vi "Actor Core.vi"(8 "error in":errorcluster, 11 "CS++DCPwrGui.lvclass":refnum<class "CS++FgenGui.lvclass">) -> (0 "error out":errorcluster, 3 "Actor out":refnum<class "Actor.lvclass">)   [LabVIEW 2013, in "CS++FgenGui.lvlib" / "CS++FgenGui.lvclass"]
doc: "(<B>Filename</B>: Actor Framework.lvlib:Actor.lvclass:Actor Core.vi)\n\nReceives messages to the actor, reacts to them, and initiates any error handling that may shut the actor down.\n\nDescendant classes may override this VI to append parallel tasks for the actor to complete while it handles messages. Overrides use the Call Parent Method node."
uses:
  CS++FgenGui.lvclass
  <vilib>/ActorFramework/Actor/Actor.lvclass
  Core/Classes/CS++ProcessVariables/ProcessVariable/PV.lvclass
  Core/Actors/CS++SVMonitor/CS++SVMonitor.lvclass
  CS++DCPwrGui Messages/Update PV Msg/Update PV Msg.lvclass
  Core/Actors/CS++BaseActor/CS++BaseActor.lvclass/CS++BaseActor.ctl
  <vilib>/ActorFramework/Actor/Actor.lvclass/Actor.ctl
  <vilib>/ActorFramework/Message Enqueuer/Message Enqueuer.lvclass/Message Enqueuer.ctl
  Core/Actors/CS++DeviceGUIActor/CS++DeviceGUIActor.lvclass/CS++DeviceGUIActor.ctl
  Core/Classes/CS++BaseClasses/Factory/CS++Factory.lvclass
  Core/Actors/CS++PVMonitor/CS++PVMonitor.lvclass/CS++PVMonitor.ctl
  Core/Actors/CS++GUIActor/CS++GUIActor.lvclass/CS++GUIActor.ctl
  Core/Actors/CS++PVMonitor Messages/Register PVs Msg/Register PVs Msg.lvclass/Register PVs Msg.ctl
  CS++FgenGui.lvclass/CS++FgenGui.ctl
  Core/Actors/CS++DeviceGUIActor/CS++DeviceGUIActor.lvclass
  Core/Classes/CS++ProcessVariables/ProcessVariable/PV.lvclass/PV.ctl
  CS++DCPwr Messages/Configure Output Enable Msg/Configure Output Enable Msg.lvclass/Configure Output Enable Msg.ctl
  CS++DCPwr Messages/Configure Output Range Msg/Configure Output Range Msg.lvclass/Configure Output Range Msg.ctl
  CS++DCPwr Messages/Configure Current Limit Msg/Configure Current Limit Msg.lvclass/Configure Current Limit Msg.ctl
  CS++DCPwr Messages/Query Max Voltage Level Msg/Query Max Voltage Level Msg.lvclass/Query Max Voltage Level Msg.ctl
  CS++DCPwr Messages/Configure OVP Msg/Configure OVP Msg.lvclass/Configure OVP Msg.ctl
  CS++DCPwr Messages/Query Max Current Limit Msg/Query Max Current Limit Msg.lvclass/Query Max Current Limit Msg.ctl
  CS++DCPwr Messages/Configure Trigger Source [TRG] Msg/Configure Trigger Source [TRG] Msg.lvclass/Configure Trigger Source [TRG] Msg.ctl
  CS++DCPwr Messages/Configure Triggered Voltage Level [TRG] Msg/Configure Triggered Voltage Level [TRG] Msg.lvclass/Configure Triggered Voltage Level [TRG] Msg.ctl
  CS++DCPwr Messages/Configure Triggered Current Limit [TRG] Msg/Configure Triggered Current Limit [TRG] Msg.lvclass/Configure Triggered Current Limit [TRG] Msg.ctl
  CS++DCPwr Messages/Configure Voltage Level Msg/Configure Voltage Level Msg.lvclass/Configure Voltage Level Msg.ctl
  Core/Actors/CS++DeviceGUIActor/Read Resource Name.vi
  Core/Actors/CS++DeviceGUIActor/Read Driver Revision.vi
  Core/Actors/CS++DeviceGUIActor/Read Firmware Revision.vi
  Core/Actors/CS++DeviceGUIActor/Read Self-Test Result Code.vi
  Core/Actors/CS++DeviceGUIActor/Read Self-Test Result Message.vi
  Core/Classes/CS++ProcessVariables/ProcessVariable/Read Data.vi
  Core/Classes/CS++ProcessVariables/ProcessVariable/Read Timestamp.vi
  <vilib>/ActorFramework/Message Enqueuer/Init from Existing Queue.vi
  <vilib>/ActorFramework/Message Enqueuer/Enqueue.vi
  <vilib>/ActorFramework/Message Priority Queue/Priority Enqueue.vi
  <vilib>/ActorFramework/Message Enqueuer/Message Enqueuer.lvclass
  Core/Actors/CS++PVMonitor Messages/CS++PVUpdate Msg/CS++PVUpdate Msg.lvclass
  Core/Actors/CS++PVMonitor Messages/Register PVs Msg/Register PVs Msg.lvclass
  <vilib>/ActorFramework/Stop Msg/Stop Msg.lvclass
  CS++DCPwr Messages/Configure Output Enable Msg/Configure Output Enable Msg.lvclass
  CS++DCPwr Messages/Configure Output Range Msg/Configure Output Range Msg.lvclass
  CS++DCPwr Messages/Configure Current Limit Msg/Configure Current Limit Msg.lvclass
  CS++DCPwr Messages/Query Max Voltage Level Msg/Query Max Voltage Level Msg.lvclass
  CS++DCPwr Messages/Configure OVP Msg/Configure OVP Msg.lvclass
  CS++DCPwr Messages/Query Max Current Limit Msg/Query Max Current Limit Msg.lvclass
  CS++DCPwr Messages/Configure Trigger Source [TRG] Msg/Configure Trigger Source [TRG] Msg.lvclass
  CS++DCPwr Messages/Configure Triggered Voltage Level [TRG] Msg/Configure Triggered Voltage Level [TRG] Msg.lvclass
  CS++DCPwr Messages/Configure Triggered Current Limit [TRG] Msg/Configure Triggered Current Limit [TRG] Msg.lvclass
  CS++DCPwr Messages/Configure Voltage Level Msg/Configure Voltage Level Msg.lvclass
  CS++DCPwr Messages/Initiate [TRG] Msg/Initiate [TRG] Msg.lvclass
  CS++DCPwr Messages/Send Software Trigger [SWT] Msg/Send Software Trigger [SWT] Msg.lvclass
  CS++DCPwr Messages/Abort [TRG] Msg/Abort [TRG] Msg.lvclass
  Core/Actors/CS++BaseActor/CS++BaseActor.lvclass
  Core/Actors/CS++GUIActor/CS++GUIActor.lvclass
  Core/Actors/CS++PVMonitor/CS++PVMonitor.lvclass
panel:
  in  "Tab Control":enum32{"Info", "Configuration", "Output"}(tab)
  out "Actor Name":string
  out "Driver Revision":string
  out "Firmware Revision":string
  out "Self-Test Result Code":i32
  out "Self-Test Result Message":string
  out "Resource Name":string
  out "Number Of Channels":i32
  in  "Configuration Settings":string[][](table)
  in  "Initiate":bool
  in  "Send Software Trigger":bool
  in  "Abort":bool
  out "Timestamp":timestamp
  in  "Stop Button":bool
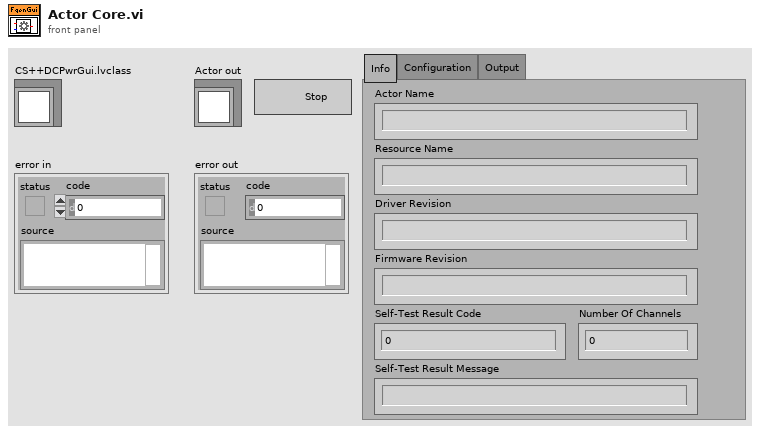
[diagram p1: front panel]
types:
  T1 = enum32{"Invalid", "Standard", "Closed", "Hidden", "Minimized", "Maximized"}
  T2 = cluster{string, "CS++FgenGui.lvlib:Update PV Msg.lvclass":refnum<class "Update PV Msg.lvclass">}
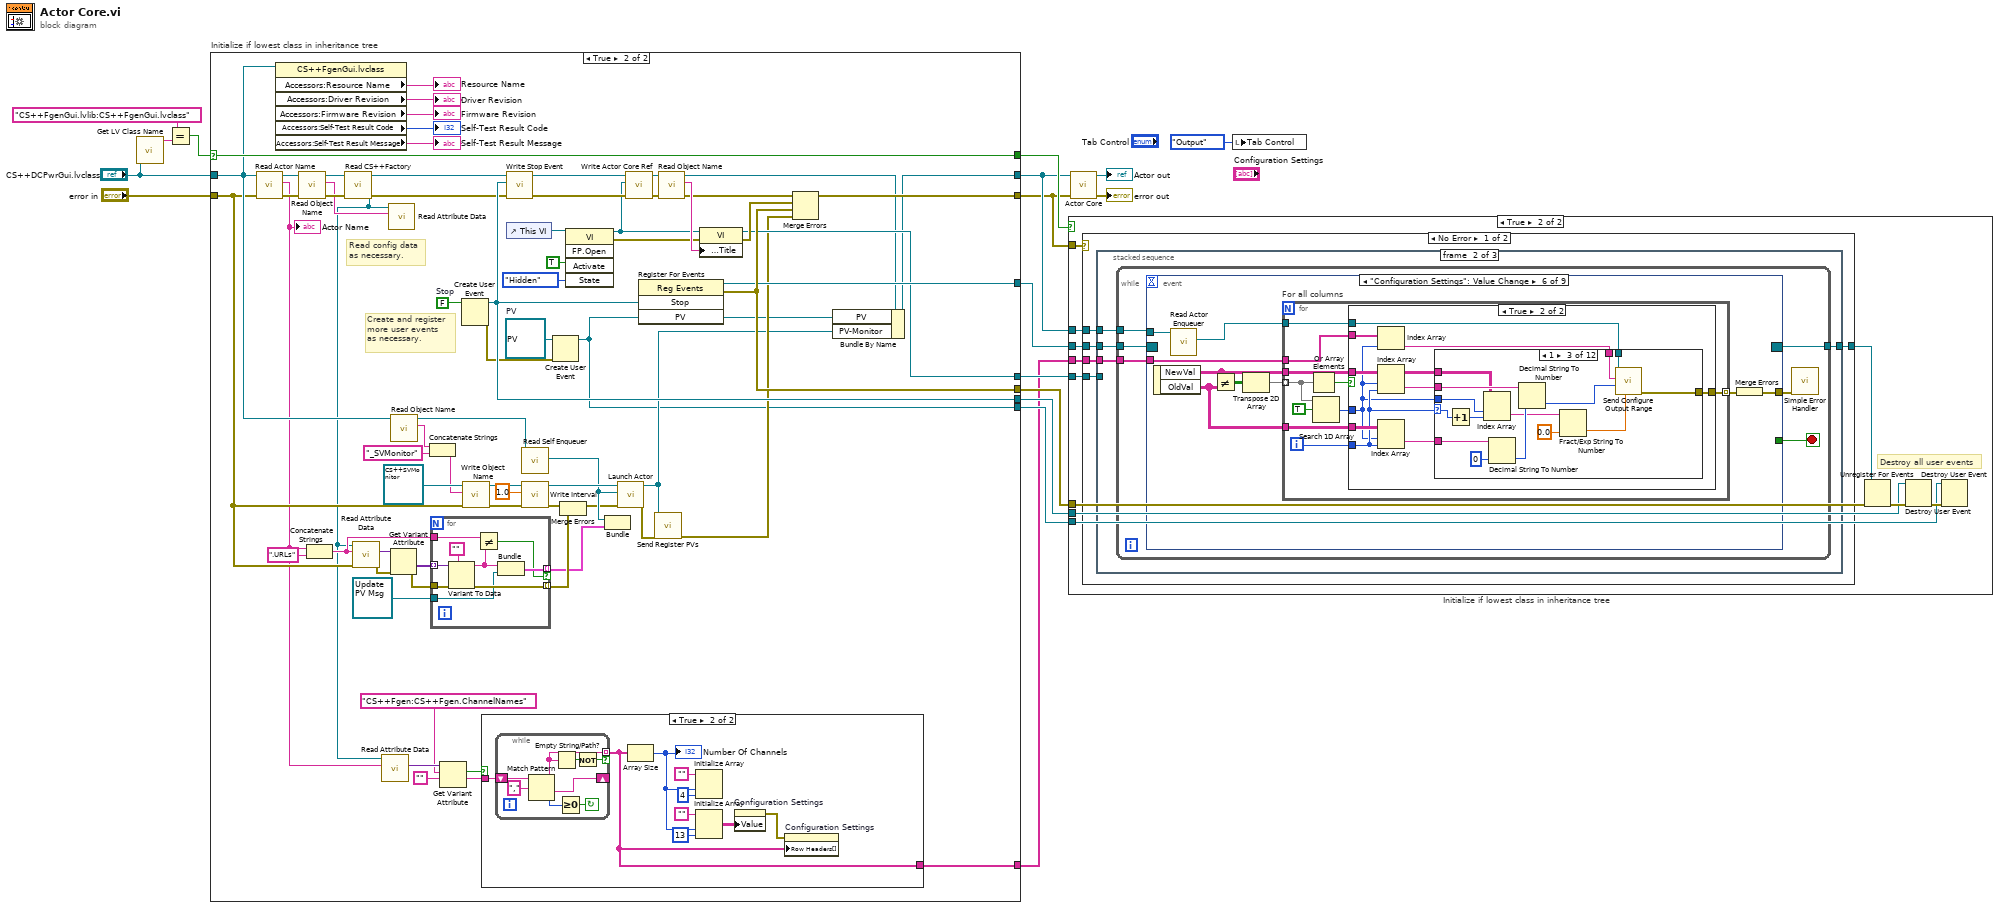
[diagram p0: block diagram]
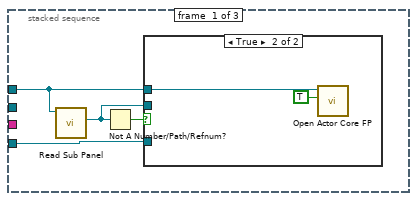
[diagram p5: hidden frame]
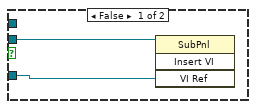
[diagram p6: hidden frame]
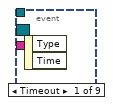
[diagram p7: hidden frame]
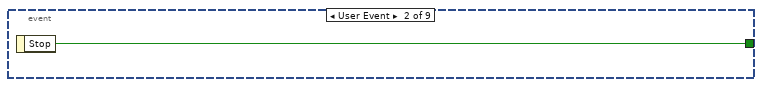
[diagram p8: hidden frame]
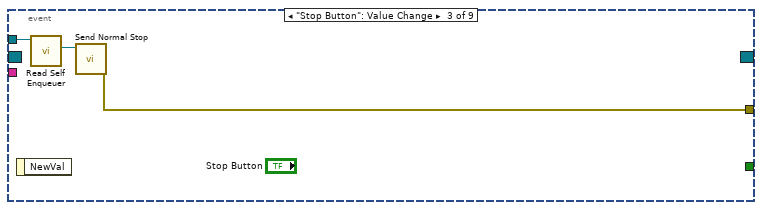
[diagram p9: hidden frame]
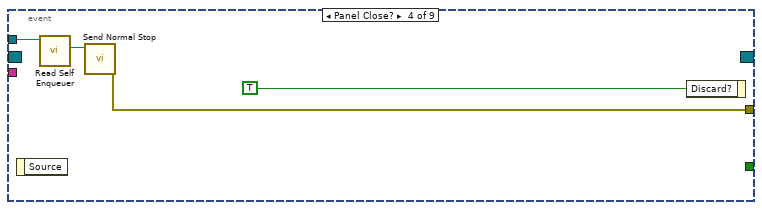
[diagram p10: hidden frame]
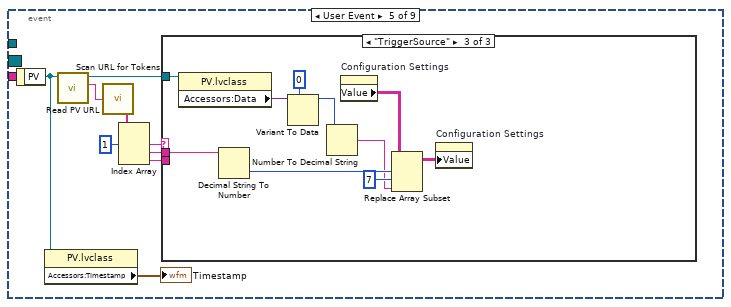
[diagram p11: hidden frame]
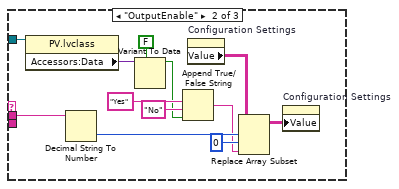
[diagram p13: hidden frame]
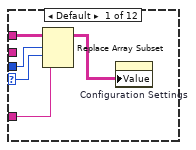
[diagram p15: hidden frame]
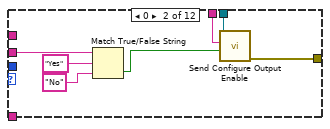
[diagram p16: hidden frame]
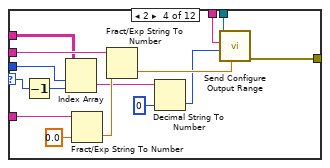
[diagram p17: hidden frame]
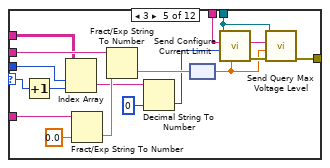
[diagram p18: hidden frame]
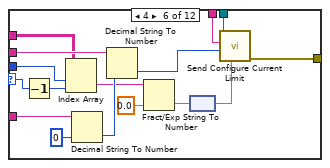
[diagram p19: hidden frame]
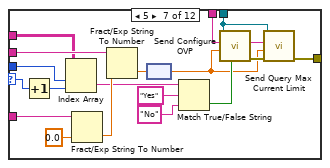
[diagram p20: hidden frame]
diagram:
  n1 = call <vilib>:"Get LV Class Name.vi"("object"="CS++DCPwrGui.lvclass") -> ("class name"=w15:string)  [unwired: 9 in, 1 out]
  n2 = Equal?(x="CS++FgenGui.lvlib:CS++FgenGui.lvclass" ("class name"), y=w15) -> (x = y?=w9:bool)
  n3 = case "Initialize if lowest class in inheritance tree" shown="True" w9 {
    selector: w9 -> [w18 w68]
    tunnel: [w19 w90] -> w4
    tunnel: "error in" -> [w19 w54]
    tunnel: [w20 w58] -> w5
    tunnel: "CS++DCPwrGui.lvclass" -> [w20 w57]
    tunnel: [_ w83] -> w13
    tunnel: [_ w82] -> w12
    tunnel: [_ w60] -> w11
    tunnel: [_ w75] -> w10
    tunnel: [w18 w68] -> w8
    tunnel: [_ w53] -> w3
    tunnel: [_ w22] -> w1
    frame False {
    }
    frame True {
      w52 = refnum<class "PV.lvclass"> refnum  # PV
      w85 = FALSE  # Stop
      # "Create and register \nmore user events\nas necessary."
      # "Read config data\nas necessary."
      n4 = call "Read Actor Name.vi"("error in (no error)"=w54, "CS++GUIActor in"=w57) -> ("error out"=w76:errorcluster, "Actor Name"=w28:string, "CS++GUIActor out"=w77:refnum<class "CS++FgenGui.lvclass">)  [unwired: 7 in]
      "Actor Name" <- w28
      n5 = property class="CS++FgenGui.lvclass"(reference=w57) -> ("Accessors:Resource Name"=→"Resource Name":string, "Accessors:Driver Revision"=→"Driver Revision":string, "Accessors:Firmware Revision"=→"Firmware Revision":string, "Accessors:Self-Test Result Code"=→"Self-Test Result Code":i32, "Accessors:Self-Test Result Message"=→"Self-Test Result Message":string)  [unwired: 1 in, 2 out]
      n6 = call "Read Object Name.vi"("error in (no error)"=w76, "CS++BaseActor in"=w77) -> ("error out"=w79:errorcluster, "Object Name"=w78:string, "CS++BaseActor out"=w80:refnum<class "CS++FgenGui.lvclass">)  [unwired: 7 in]
      n7 = Concatenate Strings(w28, ".URLs" ("string")) -> (w36:string)
      n8 = call "Read CS++Factory.vi"("error in (no error)"=w79, "CS++BaseActor in"=w80) -> ("error out"=w74:errorcluster, "CS++Factory"=w29:refnum<class "CS++Factory.lvclass">, "CS++BaseActor out"=w67:refnum<class "CS++FgenGui.lvclass">)  [unwired: 7 in]
      n9 = call-dynamic "Read Attribute Data.vi"("error in (no error)"=w54, "Object Name"=w36, "CS++Factory in"=w29) -> ("error out"=w30:errorcluster, "Attribute Data"=w31:variant)  [unwired: 6 in, 1 out]
      n10 = call-dynamic "Read Attribute Data.vi"("Object Name"=w28, "CS++Factory in"=w29) -> ("Attribute Data"=w27:variant)  [unwired: 7 in, 2 out]
      n11 = call-dynamic "Read Attribute Data.vi"("Object Name"=w78, "CS++Factory in"=w29) -> ()  [unwired: 7 in, 3 out]
      n12 = Get Variant Attribute(Variant=w31, error in=w30) -> (values=w37:variant[], error out=w38:errorcluster)  [unwired: 2 in, 2 out]
      n13 = call "Read Object Name.vi"("CS++BaseActor in"=w57) -> ("Object Name"=w43:string, "CS++BaseActor out"=w42:refnum<class "CS++FgenGui.lvclass">)  [unwired: 8 in, 1 out]
      n14 = Concatenate Strings(w43, "_SVMonitor" ("Object Name")) -> (w47:string)
      n15 = for {
        tunnel: [w116] -> w32 mode=indexing if=w112
        tunnel: w37 -> [w115] mode=indexing
        tunnel: w38 -> [w114]
        tunnel: w36 -> [w113]
        tunnel: [w109] -> w33 mode=indexing
        tunnel: refnum<class "Update PV Msg.lvclass"> refnum ("CS++FgenGui.lvlib:Update PV Msg.lvclass") -> [w108]
        n16 = Variant To Data(error in=w114, type="", Variant=w115) -> (data=w110:string, error out=w109:errorcluster)
        n17 = Not Equal?(x=w113, y=w110) -> (x != y?=w112:bool)
        n18 = Bundle(w110, "CS++FgenGui.lvlib:Update PV Msg.lvclass"=w108) -> (w116:T2)  [unwired: 1 in]
      }
      n19 = Get Variant Attribute(Variant=w27, name="CS++Fgen:CS++Fgen.ChannelNames", default value (empty Variant)="") -> (found=w24:bool, value=w23:string)  [unwired: 1 in, 2 out]
      n20 = Create User Event(user event datatype=w85) -> (user event=w75:refnum<user-event>, error out=w51:errorcluster)  [unwired: 1 in]
      n21 = call "Write Object Name.vi"("error in (no error)"=w54, "Object Name"=w47, "CS++BaseActor in"=refnum<class "CS++SVMonitor.lvclass"> refnum ("CS++SVMonitor.lvlib:CS++SVMonitor.lvclass")) -> ("error out"=w50:errorcluster, "CS++BaseActor out"=w48:refnum<class "CS++SVMonitor.lvclass">)  [unwired: 7 in]
      n22 = case shown="True" w24 {
        tunnel: w23 -> [_ w99]
        tunnel: [_ w91] -> w22
        frame False {
        }
        frame True {
          n23 = while {
            shift-right: [w105] -> _
            shift-left: w99 -> [w107]
            tunnel: [w101] -> w91 mode=indexing if=w100
            stop <- w103 continue-if-true
            n24 = Match Pattern(string=w107, regular expression=",") -> (before substring=w101:string, after substring=w105:string, offset past match=w104:i32)  [unwired: 1 in, 1 out]
            n25 = Empty String/Path?(string/path=w101) -> (empty?=w102:bool)
            n26 = Greater Or Equal To 0?(x=w104) -> (x >= 0?=w103:bool)
            n27 = Not(x=w102) -> (.not. x?=w100:bool)
          }
          n28 = Array Size(array=w91) -> (size(s)=w93:i32)
          "Number Of Channels" <- w93
          n29 = Initialize Array("", w93, 4 ("dimension size")) -> ()  [unwired: 1 out]
          n30 = Initialize Array("", w93, 13 ("dimension size")) -> (w94:string[][])
          n31 = property on="Configuration Settings" class="Tbl (strict)"("Value"=w94) -> (error out=w92:errorcluster)  [unwired: 2 in, 1 out]
          n32 = property on="Configuration Settings" class="Tbl (strict)"(error in=w92, "Row Headers[]"=w91) -> ()  [unwired: 1 in, 2 out]
        }
      }
      n33 = call "Write Stop Event.vi"("error in (no error)"=w74, "Stop"=w75, "CS++GUIActor in"=w67) -> ("error out"=w72:errorcluster, "CS++GUIActor out"=w73:refnum<class "CS++FgenGui.lvclass">)  [unwired: 7 in]
      n34 = control-ref of="This VI"() -> (w89:refnum<vi>)
      n35 = call <vilib>:"Read Self Enqueuer.vi"("Actor"=w42) -> ("Self Enqueuer"=w41:refnum<class "Message Enqueuer.lvclass">)  [unwired: 10 in]
      n36 = call "Write Interval.vi"("error in (no error)"=w50, "Interval"=dbl[unit] 1.0, "CS++PVMonitor in"=w48) -> ("error out"=w35:errorcluster, "CS++PVMonitor out"=w46:refnum<class "CS++SVMonitor.lvclass">)  [unwired: 7 in]
      n37 = Create User Event(user event datatype=w52, error in=w51) -> (user event=w53:refnum<user-event>)  [unwired: 1 out]
      n38 = Merge Errors(w35, w33) -> (w34:errorcluster)
      n39 = invoke class="VI" method="FP.Open"(reference=w89, "Activate"=TRUE ("Activate?"), "State"=T1."Hidden") -> (reference out=w61:refnum<vi>, error out=w81:errorcluster)  [unwired: 2 in, 3 out]
      n40 = Bundle("Self Enqueuer"=w41, w32) -> ()  [unwired: 1 in, 1 out]
      n41 = call <vilib>:"Launch Actor.vi"("error in (no error)"=w34, "Actor-to-Caller Enqueuer"=w41, "Actor"=w46) -> ("error out"=w40:errorcluster, "Caller-To-Actor Enqueuer"=w55:refnum<class "Message Enqueuer.lvclass">)  [unwired: 7 in]
      n42 = call "Write Actor Core Ref.vi"("error in (no error)"=w72, "Actor Core Ref"=w61, "CS++BaseActor in"=w73) -> ("error out"=w71:errorcluster, "CS++BaseActor out"=w70:refnum<class "CS++FgenGui.lvclass">)  [unwired: 7 in]
      n43 = register-events(w75, w53) -> (reference out=w82:refnum<event-registration>, error out=w83:errorcluster)  [unwired: 2 in]
      n44 = call "Send Register PVs.vi"("error in (no error)"=w40, "Message Enqueuer"=w55) -> ("error out"=w56:errorcluster)  [unwired: 8 in, 1 out]
      n45 = call "Read Object Name.vi"("error in (no error)"=w71, "CS++BaseActor in"=w70) -> ("error out"=w69:errorcluster, "Object Name"=w86:string, "CS++BaseActor out"=w59:refnum<class "CS++FgenGui.lvclass">)  [unwired: 7 in]
      n46 = property class="VI"(reference=w61, error in=w81, "Front Panel.Title"=w86) -> (reference out=w60:refnum<vi>, error out=w84:errorcluster)
      n47 = Merge Errors(w69, w84, w83, w56) -> (w90:errorcluster)
      n48 = Bundle By Name(cluster=w59, "PV"=w53, "PV-Monitor"=w55) -> (w58:refnum<class "CS++FgenGui.lvclass">)
    }
  }
  n49 = case "Initialize if lowest class in inheritance tree" shown="True" w8 {
    tunnel: w4 -> [_ w127]
    tunnel: w5 -> [_ w126]
    tunnel: w13 -> [_ w124]
    tunnel: w12 -> [_ w123]
    tunnel: w11 -> [_ w121]
    tunnel: w10 -> [_ w120]
    tunnel: w3 -> [_ w118]
    tunnel: w1 -> [_ w117]
    frame False {
    }
    frame True {
      # "Destroy all user events"
      n50 = case shown="No Error" w127 {
        tunnel: w126 -> [w132 _]
        tunnel: w123 -> [w131 w371]
        tunnel: [w130 w371] -> w122
        tunnel: w121 -> [w129 _]
        tunnel: w117 -> [w128 _]
        frame No Error {
          n51 = stacked-sequence {
            tunnel: w132 -> [w134 w143 w370]
            tunnel: w131 -> [_ w144 _]
            tunnel: [_ w142 _] -> w130
            tunnel: w129 -> [w135 _ _]
            tunnel: w128 -> [_ w141 _]
            frame #0 {
              n52 = call "Read Sub Panel.vi"("CS++GUIActor in"=w134) -> ("Sub Panel"=w133:refnum<vi>)  [unwired: 8 in, 2 out]
              n53 = Not A Number/Path/Refnum?(number/path/refnum=w133) -> (NaN/Path/Refnum?=w136:bool)
              n54 = case shown="True" w136 {
                tunnel: w134 -> [_ w140]
                tunnel: w133 -> [w138 _]
                tunnel: w135 -> [w137 _]
                frame False {
                  n55 = invoke class="SubPnl" method="Insert VI"(reference=w138, "VI Ref"=w137) -> ()  [unwired: 2 in, 4 out]
                }
                frame True {
                  n56 = call "Open Actor Core FP.vi"("Open FP (F)"=TRUE, "CS++BaseActor in"=w140) -> ()  [unwired: 8 in, 2 out]
                }
              }
            }
            frame #1 {
              n57 = while {
                tunnel: w144 -> [w150]
                tunnel: w143 -> [w149]
                tunnel: [w147] -> w142
                tunnel: w141 -> [w145]
                stop <- w148 stop-if-true
                n58 = event shown="[5] \"Configuration Settings\": Value Change" {
                  selector: w150 -> [_ _ _ _ _ _ _ _ _]
                  dyn-events: [_ _ _ _ _ _ _ _ _] -> w147
                  timeout: _ -> [_ _ _ _ _ _ _ _ _]
                  tunnel: w149 -> [_ _ w154 w156 _ w198 w362 w365 w368]
                  tunnel: [_ w151 _ _ _ _ _ _ _] -> w148
                  tunnel: [_ _ w152 w155 _ w192 w360 w363 w366] -> w146
                  tunnel: w145 -> [_ _ _ _ _ w190 _ _ _]
                  event Timeout {
                    n59 = event-data() -> ()  [unwired: 1 in, 2 out]
                  }
                  event User Event {
                    n60 = event-data() -> ("Stop"=w151:bool)  [unwired: 1 in]
                  }
                  event "Stop Button": Value Change {
                    n61 = event-data() -> ()  [unwired: 1 in, 1 out]
                    n62 = call <vilib>:"Read Self Enqueuer.vi"("Actor"=w154) -> ("Self Enqueuer"=w153:refnum<class "Message Enqueuer.lvclass">)  [unwired: 10 in]
                    n63 = call <vilib>:"Send Normal Stop.vi"("Message Enqueuer"=w153) -> ("error out"=w152:errorcluster)  [unwired: 10 in]
                  }
                  event Panel Close? {
                    n64 = event-data() -> ()  [unwired: 1 in, 1 out]
                    n65 = call <vilib>:"Read Self Enqueuer.vi"("Actor"=w156) -> ("Self Enqueuer"=w157:refnum<class "Message Enqueuer.lvclass">)  [unwired: 10 in]
                    n66 = call <vilib>:"Send Normal Stop.vi"("Message Enqueuer"=w157) -> ("error out"=w155:errorcluster)  [unwired: 10 in]
                    n67 = event-data("Discard?"=TRUE) -> ()  [unwired: 1 in, 1 out]
                  }
                  event User Event {
                    n68 = event-data() -> ("PV"=w160:refnum<class "PV.lvclass">)  [unwired: 1 in]
                    n69 = property class="PV.lvclass"(reference=w160) -> ("Accessors:Timestamp"=→"Timestamp":timestamp)  [unwired: 1 in, 2 out]
                    n70 = call "Read PV URL.vi"("PV in"=w160) -> ("PV URL"=w166:string, "PV out"=w167:refnum<class "PV.lvclass">)  [unwired: 8 in, 1 out]
                    n71 = call "Scan URL for Tokens.vi"("URL"=w166) -> ("Tokens"=w165:string[])
                    n72 = Index Array(array=w165, index #1=1 ("index")) -> (element #1=w163:string, element #2=w162:string, element #3=w161:string)  [unwired: 2 in]
                    n73 = case shown="\"TriggerSource\"" w163 {
                      tunnel: w167 -> [_ w177 w187]
                      tunnel: w162 -> [_ w172 w182]
                      tunnel: w161 -> [_ _ _]
                      frame Default {
                      }
                      frame "OutputEnable" {
                        n74 = property class="PV.lvclass"(reference=w177) -> ("Accessors:Data"=w178:variant)  [unwired: 1 in, 2 out]
                        n75 = Decimal String To Number(string=w172) -> (number=w175:i32)  [unwired: 2 in, 1 out]
                        n76 = Variant To Data(type=FALSE, Variant=w178) -> (data=w169:bool)  [unwired: 1 in, 1 out]
                        n77 = Append True/False String(1:w169, 2:"No" ("false string"), 3:"Yes" ("true string")) -> (0:w168:string)  [unwired: 1 in]
                        n78 = property on="Configuration Settings" class="Tbl (strict)"() -> ("Value"=w176:string[][])  [unwired: 2 in, 2 out]
                        n79 = Replace Array Subset(array=w176, new element=w168, index (row)=w175, index (col)=i16 0 ("precision (6)")) -> (w174:string[][])
                        n80 = property on="Configuration Settings" class="Tbl (strict)"("Value"=w174) -> ()  [unwired: 2 in, 2 out]
                      }
                      frame "TriggerSource" {
                        n81 = property class="PV.lvclass"(reference=w187) -> ("Accessors:Data"=w188:variant)  [unwired: 1 in, 2 out]
                        n82 = Decimal String To Number(string=w182) -> (number=w185:i32)  [unwired: 2 in, 1 out]
                        n83 = Variant To Data(type=0, Variant=w188) -> (data=w181:i32)  [unwired: 1 in, 1 out]
                        n84 = Number To Decimal String(number=w181) -> (decimal integer string=w180:string)  [unwired: 1 in]
                        n85 = property on="Configuration Settings" class="Tbl (strict)"() -> ("Value"=w186:string[][])  [unwired: 2 in, 2 out]
                        n86 = Replace Array Subset(array=w186, new element=w180, index (row)=w185, index (col)=i16 7 ("precision (6)")) -> (w184:string[][])
                        n87 = property on="Configuration Settings" class="Tbl (strict)"("Value"=w184) -> ()  [unwired: 2 in, 2 out]
                      }
                    }
                  }
                  event "Configuration Settings": Value Change {
                    n88 = event-data() -> ("NewVal"=w195:string[][], "OldVal"=w194:string[][])  [unwired: 1 in]
                    n89 = call "Read Actor Enqueuer.vi"("CS++GUIActor in"=w198) -> ("Actor Enqueuer"=w197:refnum<class "Message Enqueuer.lvclass">)  [unwired: 8 in, 2 out]
                    n90 = Not Equal?(x=w195, y=w194) -> (x != y?=w193:bool[][])
                    n91 = Transpose 2D Array(2D array=w193) -> (transposed array=w191:bool[][])
                    n92 = for "For all columns" {
                      tunnel: w197 -> [w208]
                      tunnel: [w207] -> w196 mode=indexing
                      tunnel: w195 -> [w206]
                      tunnel: w194 -> [w205]
                      tunnel: w191 -> [w201] mode=indexing
                      tunnel: w190 -> [w199]
                      i -> [w200]
                      n93 = Or Array Elements(Boolean array=w201) -> (logical OR=w202:bool)
                      n94 = Search 1D Array(1D array=w201, element=TRUE) -> (index of element=w203:i32)  [unwired: 1 in]
                      n95 = case shown="True" w202 {
                        tunnel: w208 -> [_ w218]
                        tunnel: [_ w217] -> w207
                        tunnel: w206 -> [_ w211]
                        tunnel: w205 -> [_ w213]
                        tunnel: w200 -> [_ w212]
                        tunnel: w203 -> [_ w210]
                        tunnel: w199 -> [_ w209]
                        frame False {
                        }
                        frame True {
                          n96 = Index Array(array=w209, index=w210) -> (element=w214:string)
                          n97 = Index Array(array=w211, index (row)=w210, index (col)=w212) -> (element=w216:string)
                          n98 = Index Array(array=w213, index (row)=w210, index (col)=w212) -> (element=w215:string)
                          n99 = case shown="1" w212 {
                            selector: w212 -> [w221 _ w235 w251 w271 w287 w305 w323 _ _ _ _]
                            tunnel: w218 -> [_ w229 w239 w255 w265 w282 w294 w320 w332 w338 w345 w354]
                            tunnel: [_ w228 w240 w256 w263 w281 w297 w321 w330 w336 w343 w351] -> w217
                            tunnel: w216 -> [_ w227 w245 w260 w277 w293 w311 w312 w329 w341 w350 w359]
                            tunnel: w215 -> [w220 _ w244 w259 w276 w292 w310 _ w327 w340 w349 w357]
                            tunnel: w214 -> [_ w230 w238 w254 w261 w283 w296 w319 w331 w337 w344 w353]
                            tunnel: w211 -> [w223 _ w237 w253 w273 w289 w307 w325 _ _ _ _]
                            tunnel: w210 -> [w222 _ w236 w252 w272 w288 w306 w324 _ _ _ _]
                            frame Default {
                              n100 = Replace Array Subset(array=w223, new element=w220, index (row)=w222, index (col)=w221) -> (w219:string[][])
                              n101 = property on="Configuration Settings" class="Tbl (strict)"("Value"=w219) -> ()  [unwired: 2 in, 2 out]
                            }
                            frame 0 {
                              n102 = Match True/False String(2:"No" ("false string"), 3:"Yes" ("true string"), 4:w227) -> (0:w224:bool)  [unwired: 1 out]
                              n103 = call "Send Configure Output Enable.vi"("enabled (true)"=w224, "channel name (\"CHANNEL1\")"=w230, "Message Enqueuer"=w229) -> ("error out"=w228:errorcluster)  [unwired: 7 in, 1 out]
                            }
                            frame 1 {
                              n104 = Increment(x=w235) -> (x+1=w231:i32)
                              n105 = Index Array(array=w237, index (row)=w236, index (col)=w231) -> (element=w234:string)
                              n106 = Decimal String To Number(string=w244, default (0L)=0 ("default (0 DBL)")) -> (number=w243:i32)  [unwired: 1 in, 1 out]
                              n107 = Decimal String To Number(string=w245, default (0L)=w243) -> (number=w241:i32)  [unwired: 1 in, 1 out]
                              n108 = Fract/Exp String To Number(string=w234, default (0 dbl)=0.0 ("default (0 DBL)")) -> (number=w233:dbl)  [unwired: 2 in, 1 out]
                              n109 = call "Send Configure Output Range.vi"("range (0.0)"=w233, "range type (Voltage)"=w241, "channel name (\"CHANNEL1\")"=w238, "Message Enqueuer"=w239) -> ("error out"=w240:errorcluster)  [unwired: 6 in, 1 out]
                            }
                            frame 2 {
                              n110 = Decrement(x=w251) -> (x-1=w248:i32)
                              n111 = Index Array(array=w253, index (row)=w252, index (col)=w248) -> (element=w250:string)
                              n112 = Fract/Exp String To Number(string=w259, default (0 dbl)=0.0 ("default (0 DBL)")) -> (number=w258:dbl)  [unwired: 2 in, 1 out]
                              n113 = Fract/Exp String To Number(string=w260, default (0 dbl)=w258) -> (number=w247:dbl)  [unwired: 2 in, 1 out]
                              n114 = Decimal String To Number(string=w250, default (0L)=0 ("default (0 DBL)")) -> (number=w246:i32)  [unwired: 1 in, 1 out]
                              n115 = call "Send Configure Output Range.vi"("range (0.0)"=w247, "range type (Voltage)"=w246, "channel name (\"CHANNEL1\")"=w254, "Message Enqueuer"=w255) -> ("error out"=w256:errorcluster)  [unwired: 6 in, 1 out]
                            }
                            frame 3 {
                              n116 = Increment(x=w271) -> (x+1=w268:i32)
                              n117 = Index Array(array=w273, index (row)=w272, index (col)=w268) -> (element=w270:string)
                              n118 = Fract/Exp String To Number(string=w276, default (0 dbl)=0.0 ("default (0 DBL)")) -> (number=w275:dbl)  [unwired: 2 in, 1 out]
                              n119 = Fract/Exp String To Number(string=w277, default (0 dbl)=w275) -> (number=w267:dbl)  [unwired: 2 in, 1 out]
                              n120 = Decimal String To Number(string=w270, default (0L)=0 ("default (0 DBL)")) -> (number=w266:i32)  [unwired: 1 in, 1 out]
                              n121 = node(w267) -> (w262:dbl[unit])
                              n122 = call "Send Configure Current Limit.vi"("limit (0.0 Amps)"=w262, "behavior (regulate)"=w266, "channel name (\"CHANNEL1\")"=w261, "Message Enqueuer"=w265) -> ("error out"=w264:errorcluster)  [unwired: 6 in, 1 out]
                              n123 = call "Send Query Max Voltage Level.vi"("error in (no error)"=w264, "current limit (0.0 Amps)"=w262, "channel name (\"CHANNEL1\")"=w261, "Message Enqueuer"=w265) -> ("error out"=w263:errorcluster)  [unwired: 6 in, 1 out]
                            }
                            frame 4 {
                              n124 = Decrement(x=w287) -> (x-1=w284:i32)
                              n125 = Index Array(array=w289, index (row)=w288, index (col)=w284) -> (element=w286:string)
                              n126 = Decimal String To Number(string=w292, default (0L)=0 ("default (0 DBL)")) -> (number=w291:i32)  [unwired: 1 in, 1 out]
                              n127 = Decimal String To Number(string=w293, default (0L)=w291) -> (number=w279:i32)  [unwired: 1 in, 1 out]
                              n128 = Fract/Exp String To Number(string=w286, default (0 dbl)=0.0 ("default (0 DBL)")) -> (number=w278:dbl)  [unwired: 2 in, 1 out]
                              n129 = node(w278) -> (w280:dbl[unit])
                              n130 = call "Send Configure Current Limit.vi"("limit (0.0 Amps)"=w280, "behavior (regulate)"=w279, "channel name (\"CHANNEL1\")"=w283, "Message Enqueuer"=w282) -> ("error out"=w281:errorcluster)  [unwired: 6 in, 1 out]
                            }
                            frame 5 {
                              n131 = Increment(x=w305) -> (x+1=w304:i32)
                              n132 = Index Array(array=w307, index (row)=w306, index (col)=w304) -> (element=w300:string)
                              n133 = Fract/Exp String To Number(string=w310, default (0 dbl)=0.0 ("default (0 DBL)")) -> (number=w309:dbl)  [unwired: 2 in, 1 out]
                              n134 = Fract/Exp String To Number(string=w311, default (0 dbl)=w309) -> (number=w303:dbl)  [unwired: 2 in, 1 out]
                              n135 = node(w303) -> (w295:dbl[unit])
                              n136 = Match True/False String(2:"No" ("false string"), 3:"Yes" ("true string"), 4:w300) -> (0:w299:bool)  [unwired: 1 out]
                              n137 = call "Send Configure OVP.vi"("enabled (true)"=w299, "limit (0.0 Volts)"=w295, "channel name (\"CHANNEL1\")"=w296, "Message Enqueuer"=w294) -> ("error out"=w298:errorcluster)  [unwired: 6 in, 1 out]
                              n138 = call "Send Query Max Current Limit.vi"("error in (no error)"=w298, "voltage level (0.0 Volts)"=w295, "channel name (\"CHANNEL1\")"=w296, "Message Enqueuer"=w294) -> ("error out"=w297:errorcluster)  [unwired: 6 in, 1 out]
                            }
                            frame 6 {
                              n139 = Decrement(x=w323) -> (x-1=w322:i32)
                              n140 = Index Array(array=w325, index (row)=w324, index (col)=w322) -> (element=w313:string)
                              n141 = Fract/Exp String To Number(string=w313) -> (number=w318:dbl)  [unwired: 3 in, 1 out]
                              n142 = Match True/False String(2:"No" ("false string"), 3:"Yes" ("true string"), 4:w312) -> (0:w314:bool)  [unwired: 1 out]
                              n143 = node(w318) -> (w317:dbl[unit])
                              n144 = call "Send Configure OVP.vi"("enabled (true)"=w314, "limit (0.0 Volts)"=w317, "channel name (\"CHANNEL1\")"=w319, "Message Enqueuer"=w320) -> ("error out"=w321:errorcluster)  [unwired: 6 in, 1 out]
                            }
                            frame 7 {
                              n145 = Decimal String To Number(string=w327) -> (number=w326:i32)  [unwired: 2 in, 1 out]
                              n146 = Decimal String To Number(string=w329, default (0L)=w326) -> (number=w328:i32)  [unwired: 1 in, 1 out]
                              n147 = call "Send Configure Trigger Source [TRG].vi"("source (Immediate)"=w328, "channel name (\"CHANNEL1\")"=w331, "Message Enqueuer"=w332) -> ("error out"=w330:errorcluster)  [unwired: 7 in, 1 out]
                            }
                            frame 8 {
                              n148 = Fract/Exp String To Number(string=w340, default (0 dbl)=0.0 ("default (0 DBL)")) -> (number=w339:dbl)  [unwired: 2 in, 1 out]
                              n149 = Fract/Exp String To Number(string=w341, default (0 dbl)=w339) -> (number=w335:dbl)  [unwired: 2 in, 1 out]
                              n150 = node(w335) -> (w334:dbl[unit])
                              n151 = call "Send Configure Triggered Voltage Level [TRG].vi"("triggered level (0.0 Volts)"=w334, "channel name (\"CHANNEL1\")"=w337, "Message Enqueuer"=w338) -> ("error out"=w336:errorcluster)  [unwired: 7 in, 1 out]
                            }
                            frame 9 {
                              n152 = Fract/Exp String To Number(string=w349, default (0 dbl)=0.0 ("default (0 DBL)")) -> (number=w348:dbl)  [unwired: 2 in, 1 out]
                              n153 = Fract/Exp String To Number(string=w350, default (0 dbl)=w348) -> (number=w347:dbl)  [unwired: 2 in, 1 out]
                              n154 = node(w347) -> (w342:dbl[unit])
                              n155 = call "Send Configure Triggered Current Limit [TRG].vi"("triggered limit (0.0 Amps)"=w342, "channel name (\"CHANNEL1\")"=w344, "Message Enqueuer"=w345) -> ("error out"=w343:errorcluster)  [unwired: 7 in, 1 out]
                            }
                            frame 12 {
                              n156 = Fract/Exp String To Number(string=w357, default (0 dbl)=0.0 ("default (0 DBL)")) -> (number=w356:dbl)  [unwired: 2 in, 1 out]
                              n157 = Fract/Exp String To Number(string=w359, default (0 dbl)=w356) -> (number=w358:dbl)  [unwired: 2 in, 1 out]
                              n158 = node(w358) -> (w352:dbl[unit])
                              n159 = call "Send Configure Voltage Level.vi"("level (0.0 Volts)"=w352, "channel name (\"CHANNEL1\")"=w353, "Message Enqueuer"=w354) -> ("error out"=w351:errorcluster)  [unwired: 7 in, 1 out]
                            }
                          }
                        }
                      }
                    }
                    n160 = Merge Errors(w196) -> (w192:errorcluster)
                  }
                  event "Initiate": Value Change {
                    n161 = event-data() -> ()  [unwired: 1 in, 1 out]
                    n162 = call "Read Actor Enqueuer.vi"("CS++GUIActor in"=w362) -> ("Actor Enqueuer"=w361:refnum<class "Message Enqueuer.lvclass">)  [unwired: 8 in, 2 out]
                    n163 = call "Send Initiate [TRG].vi"("Message Enqueuer"=w361) -> ("error out"=w360:errorcluster)  [unwired: 9 in, 1 out]
                  }
                  event "Send Software Trigger": Value Change {
                    n164 = event-data() -> ()  [unwired: 1 in, 1 out]
                    n165 = call "Read Actor Enqueuer.vi"("CS++GUIActor in"=w365) -> ("Actor Enqueuer"=w364:refnum<class "Message Enqueuer.lvclass">)  [unwired: 8 in, 2 out]
                    n166 = call "Send Send Software Trigger [SWT].vi"("Message Enqueuer"=w364) -> ("error out"=w363:errorcluster)  [unwired: 9 in, 1 out]
                  }
                  event "Abort": Value Change {
                    n167 = event-data() -> ()  [unwired: 1 in, 1 out]
                    n168 = call "Read Actor Enqueuer.vi"("CS++GUIActor in"=w368) -> ("Actor Enqueuer"=w367:refnum<class "Message Enqueuer.lvclass">)  [unwired: 8 in, 2 out]
                    n169 = call "Send Abort [TRG].vi"("Message Enqueuer"=w367) -> ("error out"=w366:errorcluster)  [unwired: 9 in, 1 out]
                  }
                }
                n170 = call <vilib>:"Simple Error Handler.vi"("error in (no error)"=w146) -> ()  [unwired: 4 in, 5 out]
              }
            }
            frame #2 {
              n171 = call "Open Actor Core FP.vi"("Open FP (F)"=FALSE, "CS++BaseActor in"=w370) -> ()  [unwired: 8 in, 2 out]
            }
          }
        }
        frame Error {
        }
      }
      n172 = Unregister For Events(event registration refnum=w122, error in=w124) -> (error out=w125:errorcluster)
      n173 = Destroy User Event(user event=w120, error in=w125) -> (error out=w119:errorcluster)
      n174 = Destroy User Event(user event=w118, error in=w119) -> ()  [unwired: 1 out]
    }
  }
  n175 = call-parent "Actor Core.vi"("error in"=w4, "CS++DeviceGUIActor.lvclass"=w5) -> ("error out"=→"error out":errorcluster, "Actor out"=→"Actor out":refnum<class "Actor.lvclass">)  [unwired: 8 in]
  n176 = local write "Tab Control"(enum32{"Info", "Configuration", "Output"}."Output" ("Tab Control")) -> ()
